vi "Read Lockin.vi"(1 "VISA resource name":refnum<visa-resource-name>="COM15", 2 "String":string="Confocal Parameters: Y Scan size:4.0000   X Scan size: 4.0000   Scan Rate:25.000    Scan Angle:0.000    mV to micron:41.000   Preamp bias off   Output 1:0.0000   Output 2:0.0000                           ;\r\n") -> (0 "String 2":string="Confocal Parameters: Y Scan size:4.0000   X Scan size: 4.0000   Scan Rate:25.000    Scan Angle:0.000    mV to micron:41.000   Preamp bias off   Output 1:0.0000   Output 2:0.0000                           ;\r\n;Lockin Parameters:Sensitivity: 17   Time Constant: 8   Filter Slope: 2   Frequency, Phase: 1000   100   ;\r\n;Lockin Outputs:Ch1 {Display, Ratio}: 0,0   Ch1 Output: 0   Ch1 Output {offset, expand}: 0,0   Ch2 Output {display,ratio} , output, {offset, expand}: 0,0   0   0,0   ;\r\n;Aux Outputs: Aux Out 1: 0   Aux Out 2,3,4: 0   0   0   ;\r\n;Other Lockin Parameters:ReserveMode: 1   Harmonic, sync: 1   0   Input Source: 0   Input ground, coupling, filter: 0   0   3   ;\r\n")   [LabVIEW 2013]
uses:
  <vilib>/Instr/_visa.llb/VISA Configure Serial Port (Instr).vi
panel:
  in  "delay before read (ms)":u32=100
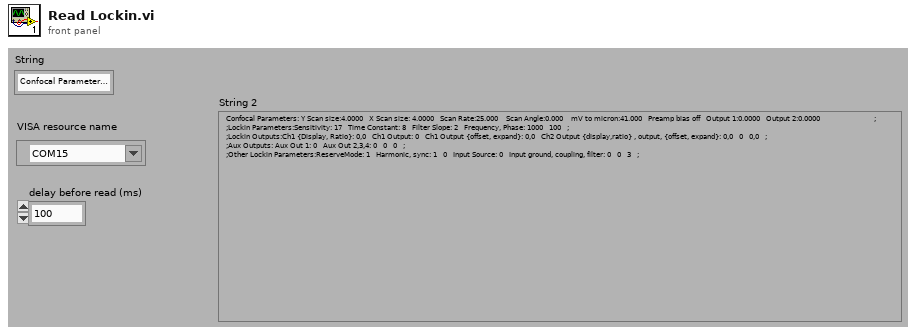
[diagram p1: front panel]
diagram:
  w57 = u16 0 items=["None"=0, "XON/XOFF"=1, "RTS/CTS"=2, "DTR/DSR"=4] ("flow control")
  w58 = u16 10 items=["1.0"=10, "1.5"=15, "2.0"=20] ("stop bits")
  w61 = u16 0 items=["None", "Odd", "Even", "Mark", "Space"] ("parity")
  w59 = FALSE  # Enable Termination Char (T)
  w60 = u32 10000  # timeout (10sec)
  # "Note:Closing the serial port allows it to be used by other applications without quitting LabVIEW."
  # "Configure Serial port (baud rate, data bits, parity, stop bits and flow control)."
  # "Close session to port."
  n1 = call-poly "VISA Configure Serial Port"("VISA resource name"="VISA resource name", "timeout (10sec)"=w60, "Enable Termination\nChar (T)"=w59, "baud rate (9600)"=u32 9600 ("baud rate"), "data bits (8)"=u16 8 ("data bits"), "parity (0:none)"=w61, "stop bits (10: 1 bit)"=w58, "flow control (0:none)"=w57) -> ("VISA resource name out"=w65:refnum<visa-resource-name>, "error out"=w66:errorcluster)  [unwired: 1 in, 5 out]
  n2 = Concatenate Strings("String", ";Lockin Parameters:" ("string")) -> (w49:string)
  n3 = flat-sequence {
    tunnel: w66 -> [w89]
    tunnel: [w74] -> w55
    tunnel: w65 -> [w88]
    tunnel: [w88] -> w54
    tunnel: [w87] -> w53
    tunnel: w49 -> [w77]
    tunnel: [w75] -> w52
    tunnel: w55 -> [w113]
    tunnel: w54 -> [w112]
    tunnel: w53 -> [_]
    tunnel: w52 -> [w100]
    tunnel: [w111] -> w45
    tunnel: [w98] -> w44
    tunnel: [w99] -> w43
    tunnel: w45 -> [w121]
    tunnel: [w119] -> w27
    tunnel: w44 -> [w122]
    tunnel: [w118] -> w26
    tunnel: w43 -> [w120]
    tunnel: [w117] -> w25
    tunnel: w27 -> [w144]
    tunnel: [w143] -> w24
    tunnel: w26 -> [w145]
    tunnel: [w142] -> w22
    tunnel: w25 -> [w146]
    tunnel: [w141] -> w20
    tunnel: w24 -> [w169]
    tunnel: [w169] -> w23
    tunnel: w22 -> [w168]
    tunnel: [w168] -> w21
    tunnel: w20 -> [w167]
    tunnel: [w165] -> w19
    tunnel: w23 -> [w175]
    tunnel: [w172] -> w36
    tunnel: w21 -> [w174]
    tunnel: [w171] -> w35
    tunnel: w19 -> [w173]
    tunnel: [w170] -> w34
    tunnel: w36 -> [w196]
    tunnel: [w197] -> w33
    tunnel: w35 -> [w195]
    tunnel: [w198] -> w32
    tunnel: w34 -> [w194]
    tunnel: [w199] -> w31
    tunnel: w33 -> [w224]
    tunnel: w32 -> [w223]
    tunnel: [w220] -> w18
    tunnel: w31 -> [w222]
    tunnel: [w221] -> w17
    tunnel: [w219] -> w16
    tunnel: w18 -> [w242]
    tunnel: [w246] -> w12
    tunnel: w17 -> [w244]
    tunnel: [w245] -> w11
    tunnel: w16 -> [w243]
    tunnel: [w247] -> w10
    tunnel: w12 -> [w273]
    tunnel: [w270] -> w9
    tunnel: w11 -> [w268]
    tunnel: [w271] -> w8
    tunnel: w10 -> [w272]
    tunnel: [w269] -> w7
    tunnel: w9 -> [w293]
    tunnel: [w296] -> w6
    tunnel: w8 -> [w294]
    tunnel: [w295] -> w4
    tunnel: w7 -> [w292]
    tunnel: [w297] -> w2
    tunnel: w6 -> [w318]
    tunnel: [w318] -> w5
    tunnel: w4 -> [w317]
    tunnel: [w317] -> w3
    tunnel: w2 -> [w316]
    tunnel: [w316] -> w1
    tunnel: w5 -> [w323]
    tunnel: [w323] -> w15
    tunnel: w3 -> [w321]
    tunnel: [w319] -> w14
    tunnel: w1 -> [w322]
    tunnel: [w322] -> w13
    tunnel: [w324] -> w42
    tunnel: w15 -> [w328]
    tunnel: [w325] -> w40
    tunnel: w14 -> [w327]
    tunnel: [w326] -> w38
    tunnel: w13 -> [w329]
    tunnel: w42 -> [w353]
    tunnel: [w350] -> w41
    tunnel: w40 -> [w352]
    tunnel: [w349] -> w39
    tunnel: w38 -> [w351]
    tunnel: [w348] -> w37
    tunnel: w41 -> [w378]
    tunnel: w39 -> [w377]
    tunnel: w37 -> [w376]
    tunnel: [w375] -> w30
    tunnel: [w374] -> w29
    tunnel: [w373] -> w28
    tunnel: [w399] -> w48
    tunnel: [w401] -> w63
    tunnel: [w400] -> w64
    tunnel: w30 -> [w396]
    tunnel: w29 -> [w397]
    tunnel: w28 -> [w398]
    frame #0 {
      # "Sensitivity"
      # "Read the number of bytes specified."
      n4 = VISA Write(VISA resource name=w88, write buffer="Sens?\n" ("string to write"), error in (no error)=w89) -> (VISA resource name out=w84:refnum<visa-resource-name>, error out=w86:errorcluster)  [unwired: 1 out]
      n5 = stacked-sequence {
        tunnel: w86 -> [w92]
        tunnel: [w92] -> w85
        tunnel: w84 -> [w91]
        tunnel: [w91] -> w83
        frame #0 {
          n6 = Wait (ms)(milliseconds to wait="delay before read (ms)") -> ()  [unwired: 1 out]
        }
      }
      n7 = property class="Instr"(reference=w83, error in=w85) -> (reference out=w82:refnum<visa-resource-name>, error out=w81:errorcluster, "Serial Settings:Number of Bytes at Serial Port"=w80:u32)
      n8 = VISA Read(VISA resource name=w82, byte count=w80, error in (no error)=w81) -> (VISA resource name out=w87:refnum<visa-resource-name>, read buffer=w70:string, error out=w74:errorcluster)  [unwired: 1 out]
      n9 = Search and Replace String(replace all?=TRUE ("replace all? (F)"), input string=w70, search string="\r", replace string="   " ("replace string (\"\")")) -> (result string=w69:string)  [unwired: 4 in, 3 out]
      n10 = Concatenate Strings("Sensitivity: ", w69) -> (w76:string)
      n11 = Concatenate Strings(w77, w76) -> (w75:string)
    }
    frame #1 {
      # "Time constant"
      # "Read the number of bytes specified."
      n12 = VISA Write(VISA resource name=w112, write buffer="OFLT?\n" ("string to write"), error in (no error)=w113) -> (VISA resource name out=w108:refnum<visa-resource-name>, error out=w110:errorcluster)  [unwired: 1 out]
      n13 = stacked-sequence {
        tunnel: w110 -> [w116]
        tunnel: [w116] -> w109
        tunnel: w108 -> [w115]
        tunnel: [w115] -> w107
        frame #0 {
          n14 = local read "delay before read (ms)"() -> (w114:u32)
          n15 = Wait (ms)(milliseconds to wait=w114) -> ()  [unwired: 1 out]
        }
      }
      n16 = property class="Instr"(reference=w107, error in=w109) -> (reference out=w106:refnum<visa-resource-name>, error out=w105:errorcluster, "Serial Settings:Number of Bytes at Serial Port"=w104:u32)
      n17 = VISA Read(VISA resource name=w106, byte count=w104, error in (no error)=w105) -> (VISA resource name out=w98:refnum<visa-resource-name>, read buffer=w94:string, error out=w111:errorcluster)  [unwired: 1 out]
      n18 = Search and Replace String(replace all?=TRUE ("replace all? (F)"), input string=w94, search string="\r", replace string="   " ("replace string (\"\")")) -> (result string=w93:string)  [unwired: 4 in, 3 out]
      n19 = Concatenate Strings("Time Constant: ", w93) -> (w101:string)
      n20 = Concatenate Strings(w100, w101) -> (w99:string)
    }
    frame #2 {
      # "Time constant"
      # "Read the number of bytes specified."
      n21 = VISA Write(VISA resource name=w122, write buffer="OFSL?\n" ("string to write"), error in (no error)=w121) -> (VISA resource name out=w125:refnum<visa-resource-name>, error out=w123:errorcluster)  [unwired: 1 out]
      n22 = stacked-sequence {
        tunnel: w123 -> [w140]
        tunnel: [w140] -> w124
        tunnel: w125 -> [w139]
        tunnel: [w139] -> w126
        frame #0 {
          n23 = local read "delay before read (ms)"() -> (w138:u32)
          n24 = Wait (ms)(milliseconds to wait=w138) -> ()  [unwired: 1 out]
        }
      }
      n25 = property class="Instr"(reference=w126, error in=w124) -> (reference out=w127:refnum<visa-resource-name>, error out=w128:errorcluster, "Serial Settings:Number of Bytes at Serial Port"=w129:u32)
      n26 = VISA Read(VISA resource name=w127, byte count=w129, error in (no error)=w128) -> (VISA resource name out=w118:refnum<visa-resource-name>, read buffer=w136:string, error out=w119:errorcluster)  [unwired: 1 out]
      n27 = Search and Replace String(replace all?=TRUE ("replace all? (F)"), input string=w136, search string="\r", replace string="   " ("replace string (\"\")")) -> (result string=w137:string)  [unwired: 4 in, 3 out]
      n28 = Concatenate Strings("Filter Slope: ", w137) -> (w132:string)
      n29 = Concatenate Strings(w120, w132) -> (w117:string)
    }
    frame #3 {
      # "Time constant"
      # "Read the number of bytes specified."
      n30 = VISA Write(VISA resource name=w145, write buffer="FREQ?\nPHAS?\n" ("string to write"), error in (no error)=w144) -> (VISA resource name out=w159:refnum<visa-resource-name>, error out=w161:errorcluster)  [unwired: 1 out]
      n31 = stacked-sequence {
        tunnel: w161 -> [w164]
        tunnel: [w164] -> w160
        tunnel: w159 -> [w163]
        tunnel: [w163] -> w158
        frame #0 {
          n32 = local read "delay before read (ms)"() -> (w162:u32)
          n33 = Wait (ms)(milliseconds to wait=w162) -> ()  [unwired: 1 out]
        }
      }
      n34 = property class="Instr"(reference=w158, error in=w160) -> (reference out=w157:refnum<visa-resource-name>, error out=w156:errorcluster, "Serial Settings:Number of Bytes at Serial Port"=w155:u32)
      n35 = VISA Read(VISA resource name=w157, byte count=w155, error in (no error)=w156) -> (VISA resource name out=w142:refnum<visa-resource-name>, read buffer=w148:string, error out=w143:errorcluster)  [unwired: 1 out]
      n36 = Search and Replace String(replace all?=TRUE ("replace all? (F)"), input string=w148, search string="\r", replace string="   " ("replace string (\"\")")) -> (result string=w147:string)  [unwired: 4 in, 3 out]
      n37 = Concatenate Strings("Frequency, Phase: ", w147) -> (w152:string)
      n38 = Concatenate Strings(w146, w152) -> (w141:string)
    }
    frame #4 {
      n39 = Concatenate Strings(w167, ";\r\n;Lockin Outputs:" ("string")) -> (w165:string)
    }
    frame #5 {
      # "Time constant"
      # "Read the number of bytes specified."
      n40 = VISA Write(VISA resource name=w174, write buffer="DDEF?1\n" ("string to write"), error in (no error)=w175) -> (VISA resource name out=w188:refnum<visa-resource-name>, error out=w190:errorcluster)  [unwired: 1 out]
      n41 = stacked-sequence {
        tunnel: w190 -> [w193]
        tunnel: [w193] -> w189
        tunnel: w188 -> [w192]
        tunnel: [w192] -> w187
        frame #0 {
          n42 = local read "delay before read (ms)"() -> (w191:u32)
          n43 = Wait (ms)(milliseconds to wait=w191) -> ()  [unwired: 1 out]
        }
      }
      n44 = property class="Instr"(reference=w187, error in=w189) -> (reference out=w186:refnum<visa-resource-name>, error out=w185:errorcluster, "Serial Settings:Number of Bytes at Serial Port"=w184:u32)
      n45 = VISA Read(VISA resource name=w186, byte count=w184, error in (no error)=w185) -> (VISA resource name out=w171:refnum<visa-resource-name>, read buffer=w177:string, error out=w172:errorcluster)  [unwired: 1 out]
      n46 = Search and Replace String(replace all?=TRUE ("replace all? (F)"), input string=w177, search string="\r", replace string="   " ("replace string (\"\")")) -> (result string=w176:string)  [unwired: 4 in, 3 out]
      n47 = Concatenate Strings("Ch1 {Display, Ratio}: ", w176) -> (w181:string)
      n48 = Concatenate Strings(w173, w181) -> (w170:string)
    }
    frame #6 {
      # "Time constant"
      # "Read the number of bytes specified."
      n49 = VISA Write(VISA resource name=w195, write buffer="FPOP?1\n" ("string to write"), error in (no error)=w196) -> (VISA resource name out=w202:refnum<visa-resource-name>, error out=w200:errorcluster)  [unwired: 1 out]
      n50 = stacked-sequence {
        tunnel: w200 -> [w217]
        tunnel: [w217] -> w201
        tunnel: w202 -> [w216]
        tunnel: [w216] -> w203
        frame #0 {
          n51 = local read "delay before read (ms)"() -> (w215:u32)
          n52 = Wait (ms)(milliseconds to wait=w215) -> ()  [unwired: 1 out]
        }
      }
      n53 = property class="Instr"(reference=w203, error in=w201) -> (reference out=w204:refnum<visa-resource-name>, error out=w205:errorcluster, "Serial Settings:Number of Bytes at Serial Port"=w206:u32)
      n54 = VISA Read(VISA resource name=w204, byte count=w206, error in (no error)=w205) -> (VISA resource name out=w198:refnum<visa-resource-name>, read buffer=w213:string, error out=w197:errorcluster)  [unwired: 1 out]
      n55 = Search and Replace String(replace all?=TRUE ("replace all? (F)"), input string=w213, search string="\r", replace string="   " ("replace string (\"\")")) -> (result string=w214:string)  [unwired: 4 in, 3 out]
      n56 = Concatenate Strings("Ch1 Output: ", w214) -> (w209:string)
      n57 = Concatenate Strings(w194, w209) -> (w199:string)
    }
    frame #7 {
      # "Time constant"
      # "Read the number of bytes specified."
      n58 = VISA Write(VISA resource name=w223, write buffer="OEXP?1\n" ("string to write"), error in (no error)=w224) -> (VISA resource name out=w236:refnum<visa-resource-name>, error out=w238:errorcluster)  [unwired: 1 out]
      n59 = stacked-sequence {
        tunnel: w238 -> [w241]
        tunnel: [w241] -> w237
        tunnel: w236 -> [w240]
        tunnel: [w240] -> w235
        frame #0 {
          n60 = local read "delay before read (ms)"() -> (w239:u32)
          n61 = Wait (ms)(milliseconds to wait=w239) -> ()  [unwired: 1 out]
        }
      }
      n62 = property class="Instr"(reference=w235, error in=w237) -> (reference out=w234:refnum<visa-resource-name>, error out=w233:errorcluster, "Serial Settings:Number of Bytes at Serial Port"=w232:u32)
      n63 = VISA Read(VISA resource name=w234, byte count=w232, error in (no error)=w233) -> (VISA resource name out=w220:refnum<visa-resource-name>, read buffer=w226:string, error out=w219:errorcluster)  [unwired: 1 out]
      n64 = Search and Replace String(replace all?=TRUE ("replace all? (F)"), input string=w226, search string="\r", replace string="   " ("replace string (\"\")")) -> (result string=w225:string)  [unwired: 4 in, 3 out]
      n65 = Concatenate Strings("Ch1 Output {offset, expand}: ", w225) -> (w230:string)
      n66 = Concatenate Strings(w222, w230) -> (w221:string)
    }
    frame #8 {
      # "Time constant"
      # "Read the number of bytes specified."
      n67 = VISA Write(VISA resource name=w242, write buffer="DDEF?2\nFPOP?2\nOEXP?2\n" ("string to write"), error in (no error)=w243) -> (VISA resource name out=w250:refnum<visa-resource-name>, error out=w248:errorcluster)  [unwired: 1 out]
      n68 = stacked-sequence {
        tunnel: w248 -> [w265]
        tunnel: [w265] -> w249
        tunnel: w250 -> [w264]
        tunnel: [w264] -> w251
        frame #0 {
          n69 = local read "delay before read (ms)"() -> (w263:u32)
          n70 = Wait (ms)(milliseconds to wait=w263) -> ()  [unwired: 1 out]
        }
      }
      n71 = property class="Instr"(reference=w251, error in=w249) -> (reference out=w252:refnum<visa-resource-name>, error out=w253:errorcluster, "Serial Settings:Number of Bytes at Serial Port"=w254:u32)
      n72 = VISA Read(VISA resource name=w252, byte count=w254, error in (no error)=w253) -> (VISA resource name out=w246:refnum<visa-resource-name>, read buffer=w260:string, error out=w247:errorcluster)  [unwired: 1 out]
      n73 = Search and Replace String(replace all?=TRUE ("replace all? (F)"), input string=w260, search string="\r", replace string="   " ("replace string (\"\")")) -> (result string=w261:string)  [unwired: 4 in, 3 out]
      n74 = Concatenate Strings("Ch2 Output {display,ratio} , output, {offset, expand}: ", w261) -> (w256:string)
      n75 = Concatenate Strings(w244, w256) -> (w245:string)
    }
    frame #9 {
      # "Time constant"
      # "Read the number of bytes specified."
      n76 = Concatenate Strings(w268, ";\r\n;Aux Outputs: " ("string")) -> (w266:string)
      n77 = VISA Write(VISA resource name=w273, write buffer="AUXV?1\n" ("string to write"), error in (no error)=w272) -> (VISA resource name out=w286:refnum<visa-resource-name>, error out=w288:errorcluster)  [unwired: 1 out]
      n78 = stacked-sequence {
        tunnel: w288 -> [w291]
        tunnel: [w291] -> w287
        tunnel: w286 -> [w290]
        tunnel: [w290] -> w285
        frame #0 {
          n79 = local read "delay before read (ms)"() -> (w289:u32)
          n80 = Wait (ms)(milliseconds to wait=w289) -> ()  [unwired: 1 out]
        }
      }
      n81 = property class="Instr"(reference=w285, error in=w287) -> (reference out=w284:refnum<visa-resource-name>, error out=w283:errorcluster, "Serial Settings:Number of Bytes at Serial Port"=w282:u32)
      n82 = VISA Read(VISA resource name=w284, byte count=w282, error in (no error)=w283) -> (VISA resource name out=w270:refnum<visa-resource-name>, read buffer=w276:string, error out=w269:errorcluster)  [unwired: 1 out]
      n83 = Search and Replace String(replace all?=TRUE ("replace all? (F)"), input string=w276, search string="\r", replace string="   " ("replace string (\"\")")) -> (result string=w275:string)  [unwired: 4 in, 3 out]
      n84 = Concatenate Strings("Aux Out 1: ", w275) -> (w280:string)
      n85 = Concatenate Strings(w266, w280) -> (w271:string)
    }
    frame #10 {
      # "Time constant"
      # "Read the number of bytes specified."
      n86 = VISA Write(VISA resource name=w293, write buffer="AUXV?2\nAUXV?3\nAUXV?3\n" ("string to write"), error in (no error)=w292) -> (VISA resource name out=w300:refnum<visa-resource-name>, error out=w298:errorcluster)  [unwired: 1 out]
      n87 = stacked-sequence {
        tunnel: w298 -> [w315]
        tunnel: [w315] -> w299
        tunnel: w300 -> [w314]
        tunnel: [w314] -> w301
        frame #0 {
          n88 = local read "delay before read (ms)"() -> (w313:u32)
          n89 = Wait (ms)(milliseconds to wait=w313) -> ()  [unwired: 1 out]
        }
      }
      n90 = property class="Instr"(reference=w301, error in=w299) -> (reference out=w302:refnum<visa-resource-name>, error out=w303:errorcluster, "Serial Settings:Number of Bytes at Serial Port"=w304:u32)
      n91 = VISA Read(VISA resource name=w302, byte count=w304, error in (no error)=w303) -> (VISA resource name out=w296:refnum<visa-resource-name>, read buffer=w310:string, error out=w297:errorcluster)  [unwired: 1 out]
      n92 = Search and Replace String(replace all?=TRUE ("replace all? (F)"), input string=w310, search string="\r", replace string="   " ("replace string (\"\")")) -> (result string=w311:string)  [unwired: 4 in, 3 out]
      n93 = Concatenate Strings("Aux Out 2,3,4: ", w311) -> (w306:string)
      n94 = Concatenate Strings(w294, w306) -> (w295:string)
    }
    frame #11 {
    }
    frame #12 {
      n95 = Concatenate Strings(w321, ";\r\n;Other Lockin Parameters:" ("string")) -> (w319:string)
    }
    frame #13 {
      # "Time constant"
      # "Read the number of bytes specified."
      n96 = VISA Write(VISA resource name=w328, write buffer="RMOD?\n" ("string to write"), error in (no error)=w329) -> (VISA resource name out=w342:refnum<visa-resource-name>, error out=w344:errorcluster)  [unwired: 1 out]
      n97 = stacked-sequence {
        tunnel: w344 -> [w347]
        tunnel: [w347] -> w343
        tunnel: w342 -> [w346]
        tunnel: [w346] -> w341
        frame #0 {
          n98 = local read "delay before read (ms)"() -> (w345:u32)
          n99 = Wait (ms)(milliseconds to wait=w345) -> ()  [unwired: 1 out]
        }
      }
      n100 = property class="Instr"(reference=w341, error in=w343) -> (reference out=w340:refnum<visa-resource-name>, error out=w339:errorcluster, "Serial Settings:Number of Bytes at Serial Port"=w338:u32)
      n101 = VISA Read(VISA resource name=w340, byte count=w338, error in (no error)=w339) -> (VISA resource name out=w325:refnum<visa-resource-name>, read buffer=w331:string, error out=w324:errorcluster)  [unwired: 1 out]
      n102 = Search and Replace String(replace all?=TRUE ("replace all? (F)"), input string=w331, search string="\r", replace string="   " ("replace string (\"\")")) -> (result string=w330:string)  [unwired: 4 in, 3 out]
      n103 = Concatenate Strings("ReserveMode: ", w330) -> (w335:string)
      n104 = Concatenate Strings(w327, w335) -> (w326:string)
    }
    frame #14 {
      # "Time constant"
      # "Read the number of bytes specified."
      n105 = VISA Write(VISA resource name=w352, write buffer="HARM?\nSYNC?\n" ("string to write"), error in (no error)=w353) -> (VISA resource name out=w356:refnum<visa-resource-name>, error out=w354:errorcluster)  [unwired: 1 out]
      n106 = stacked-sequence {
        tunnel: w354 -> [w371]
        tunnel: [w371] -> w355
        tunnel: w356 -> [w370]
        tunnel: [w370] -> w357
        frame #0 {
          n107 = local read "delay before read (ms)"() -> (w369:u32)
          n108 = Wait (ms)(milliseconds to wait=w369) -> ()  [unwired: 1 out]
        }
      }
      n109 = property class="Instr"(reference=w357, error in=w355) -> (reference out=w358:refnum<visa-resource-name>, error out=w359:errorcluster, "Serial Settings:Number of Bytes at Serial Port"=w360:u32)
      n110 = VISA Read(VISA resource name=w358, byte count=w360, error in (no error)=w359) -> (VISA resource name out=w349:refnum<visa-resource-name>, read buffer=w367:string, error out=w350:errorcluster)  [unwired: 1 out]
      n111 = Search and Replace String(replace all?=TRUE ("replace all? (F)"), input string=w367, search string="\r", replace string="   " ("replace string (\"\")")) -> (result string=w368:string)  [unwired: 4 in, 3 out]
      n112 = Concatenate Strings("Harmonic, sync: ", w368) -> (w363:string)
      n113 = Concatenate Strings(w351, w363) -> (w348:string)
    }
    frame #15 {
      # "Input Source"
      # "Read the number of bytes specified."
      n114 = VISA Write(VISA resource name=w377, write buffer="ISRC?\n" ("string to write"), error in (no error)=w378) -> (VISA resource name out=w381:refnum<visa-resource-name>, error out=w379:errorcluster)  [unwired: 1 out]
      n115 = stacked-sequence {
        tunnel: w379 -> [w395]
        tunnel: [w395] -> w380
        tunnel: w381 -> [w394]
        tunnel: [w394] -> w382
        frame #0 {
          n116 = local read "delay before read (ms)"() -> (w393:u32)
          n117 = Wait (ms)(milliseconds to wait=w393) -> ()  [unwired: 1 out]
        }
      }
      n118 = property class="Instr"(reference=w382, error in=w380) -> (reference out=w383:refnum<visa-resource-name>, error out=w384:errorcluster, "Serial Settings:Number of Bytes at Serial Port"=w385:u32)
      n119 = VISA Read(VISA resource name=w383, byte count=w385, error in (no error)=w384) -> (VISA resource name out=w374:refnum<visa-resource-name>, read buffer=w392:string, error out=w375:errorcluster)  [unwired: 1 out]
      n120 = Search and Replace String(replace all?=TRUE ("replace all? (F)"), input string=w392, search string="\r", replace string="   " ("replace string (\"\")")) -> (result string=w372:string)  [unwired: 4 in, 3 out]
      n121 = Concatenate Strings("Input Source: ", w372) -> (w388:string)
      n122 = Concatenate Strings(w376, w388) -> (w373:string)
    }
    frame #16 {
      # "Input Source"
      # "Read the number of bytes specified."
      n123 = VISA Write(VISA resource name=w397, write buffer="IGND?\n ICPL?\n ILIN?\n" ("string to write"), error in (no error)=w396) -> (VISA resource name out=w413:refnum<visa-resource-name>, error out=w415:errorcluster)  [unwired: 1 out]
      n124 = stacked-sequence {
        tunnel: w415 -> [w419]
        tunnel: [w419] -> w414
        tunnel: w413 -> [w418]
        tunnel: [w418] -> w412
        frame #0 {
          n125 = local read "delay before read (ms)"() -> (w417:u32)
          n126 = Wait (ms)(milliseconds to wait=w417) -> ()  [unwired: 1 out]
        }
      }
      n127 = property class="Instr"(reference=w412, error in=w414) -> (reference out=w411:refnum<visa-resource-name>, error out=w410:errorcluster, "Serial Settings:Number of Bytes at Serial Port"=w409:u32)
      n128 = VISA Read(VISA resource name=w411, byte count=w409, error in (no error)=w410) -> (VISA resource name out=w401:refnum<visa-resource-name>, read buffer=w402:string, error out=w400:errorcluster)  [unwired: 1 out]
      n129 = Search and Replace String(replace all?=TRUE ("replace all? (F)"), input string=w402, search string="\r", replace string="   " ("replace string (\"\")")) -> (result string=w416:string)  [unwired: 4 in, 3 out]
      n130 = Concatenate Strings("Input ground, coupling, filter: ", w416) -> (w406:string)
      n131 = Concatenate Strings(w398, w406) -> (w399:string)
    }
  }
  n132 = VISA Close(VISA resource name=w63, error in (no error)=w64) -> (error out=w62:errorcluster)
  n133 = call <vilib>:"Simple Error Handler.vi"("error in (no error)"=w62) -> ()  [unwired: 1 in, 8 out]
  n134 = Concatenate Strings(w48, ";\r\n" ("string")) -> (→"String 2":string)
